vi "getNormal&LoopParaArraySubsetEachTime.vi"(8 "paraArray":string[](array[string]), 9 "loopParaEndNum":i32=5, 10 "loopParaStartNum":i32=1, 11 "lastLoopParaEndNum":i32=5) -> (2 "loopParaArray":string[](array[string]), 3 "normalParaArray":string[](array[string]))   [LabVIEW 2010]
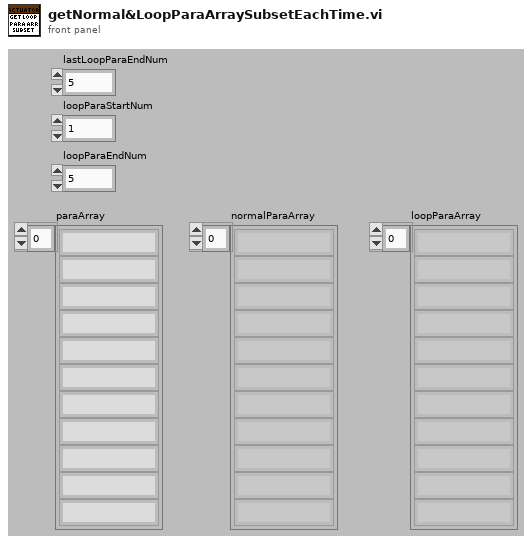
[diagram p1: front panel]
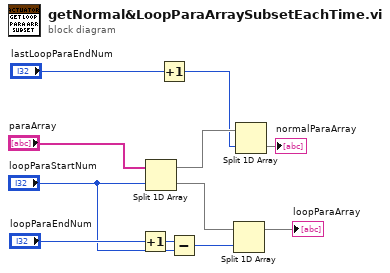
[diagram p0: block diagram]
diagram:
  n1 = Increment(x="loopParaEndNum") -> (x+1=w10:i32)
  n2 = Split 1D Array(array="paraArray", index="loopParaStartNum") -> (first subarray=w4:string[], second subarray=w7:string[])
  n3 = Increment(x="lastLoopParaEndNum") -> (x+1=w1:i32)
  n4 = Subtract(x=w10, y="loopParaStartNum") -> (x-y=w11:i32)
  n5 = Split 1D Array(array=w7, index=w11) -> (first subarray=→"loopParaArray":string[])  [unwired: 1 out]
  n6 = Split 1D Array(array=w4, index=w1) -> (second subarray=→"normalParaArray":string[])  [unwired: 1 out]
